vi "AssetInterface_Write Process Name.vi"(10 "Process Name":string, 11 "EnergyStorage in":refnum<class "EnergyStorage.lvclass">) -> (3 "EnergyStorage out":refnum<class "EnergyStorage.lvclass">)   [LabVIEW 2015, in "EnergyStorage.lvclass"]
uses:
  EnergyStorage.lvclass
  EnergyStorage.lvclass/EnergyStorage.ctl
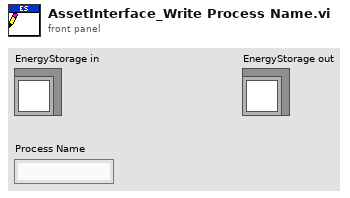
[diagram p1: front panel]
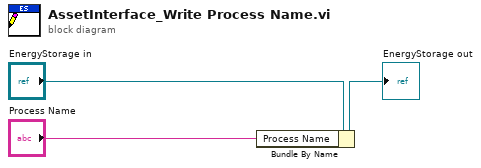
[diagram p0: block diagram]
diagram:
  n1 = Bundle By Name(cluster="EnergyStorage in", "Process Name"="Process Name") -> (→"EnergyStorage out":refnum<class "EnergyStorage.lvclass">)
